vi "New JKISM_2024 for Tests.vi"(7 "Open SM FP (for debugging)":bool, 8 "error in (no error)":errorcluster) -> (0 "error out":errorcluster, 3 "JKI SM out":refnum<class "JKI SM.lvclass">)   [LabVIEW 2020, in "JKI State Machine API - Tests.lvlib"]
uses:
  source/JKI SM/JKI SM.lvclass
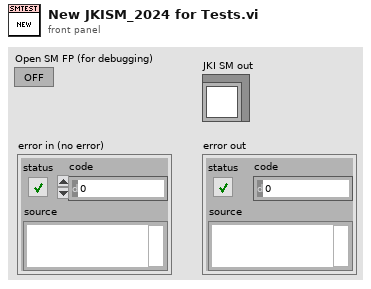
[diagram p1: front panel]
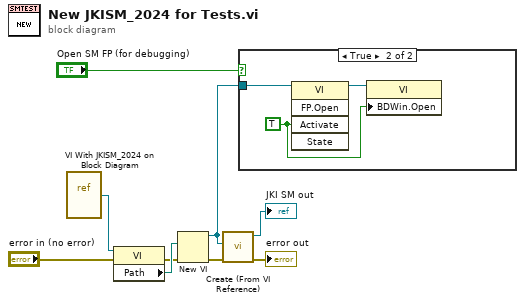
[diagram p0: block diagram]
diagram:
  n1 = vi-ref "VI With JKISM_2024 on Block Diagram.vi"() -> (w5:refnum<vi>)
  n2 = property class="VI"(reference=w5, error in="error in (no error)") -> (error out=w3:errorcluster, "Path"=w4:path)  [unwired: 1 out]
  n3 = New VI(8:w3, 10:w4) -> (0:w7:errorcluster, 3:w2:refnum<vi>)  [unwired: 5 in]
  n4 = call "Create (From VI Reference).vi"("error in (no error)"=w7, "VI"=w2) -> ("error out"=→"error out":errorcluster, "JKI SM out"=→"JKI SM out":refnum<class "JKI SM.lvclass">)  [unwired: 8 in]
  n5 = case shown="True" "Open SM FP (for debugging)" {
    tunnel: w2 -> [_ w12]
    frame False {
    }
    frame True {
      w10 = TRUE ("Activate?")
      n6 = invoke class="VI" method="FP.Open"(reference=w12, "Activate"=w10) -> (reference out=w11:refnum<vi>)  [unwired: 3 in, 4 out]
      n7 = property class="VI"(reference=w11, "BDWin.Open"=w10) -> ()  [unwired: 1 in, 2 out]
    }
  }
